vi "log_data.vi"(0 "Log File":path, 1 "Carrier amplitudes":T7 format="%#_3p", 2 "Display card":i32=1 min=0 max=3 step=1, 5 "Start Logging":bool, 7 "High carrier amplitudes":T4 format="%#_3p", 9 "Stop Logging":bool, 11 "Time Stamp":timestamp, 12 "Trace info":T1, 13 "Log mode":T5, 14 "Modulation info":T6={"Fs full"=0.0, "Fs high"=0.0, "Fs low"=0.0, "Read size"=5000, "FFT size low"=5000, "df low"=5000.0, "High carriers"=[], "Low carriers"=[], "Hi channels at low"=[7]} {"Hi channels at low" min=0 step=1; "Low carriers" format="%#_6p"; "High carriers" format="%#_6p"}) -> (4 "Logging":bool)   [LabVIEW 2014]
doc: "Converts an array of data to a row of tab-separated columns, prepends the timestamp column, and terminates each row with the end of line character."
uses:
  processing/carrier_amplitudes.ctl
  processing/modulation_info.ctl
  log_mode.ctl
  processing/high_carrier_amplitudes.ctl
  gui/trace_info.ctl
  gui/trace_channel.ctl
  main/ilemt_status.ctl
  main/ilemt_globals.vi
panel:
  out "Result string":string
  # "Debug display:"
  # "Note that each dumped row is a couping matrix in column major format, where rows are source axes and columns are sensor axes. See comment in coupling_to_string for more details."
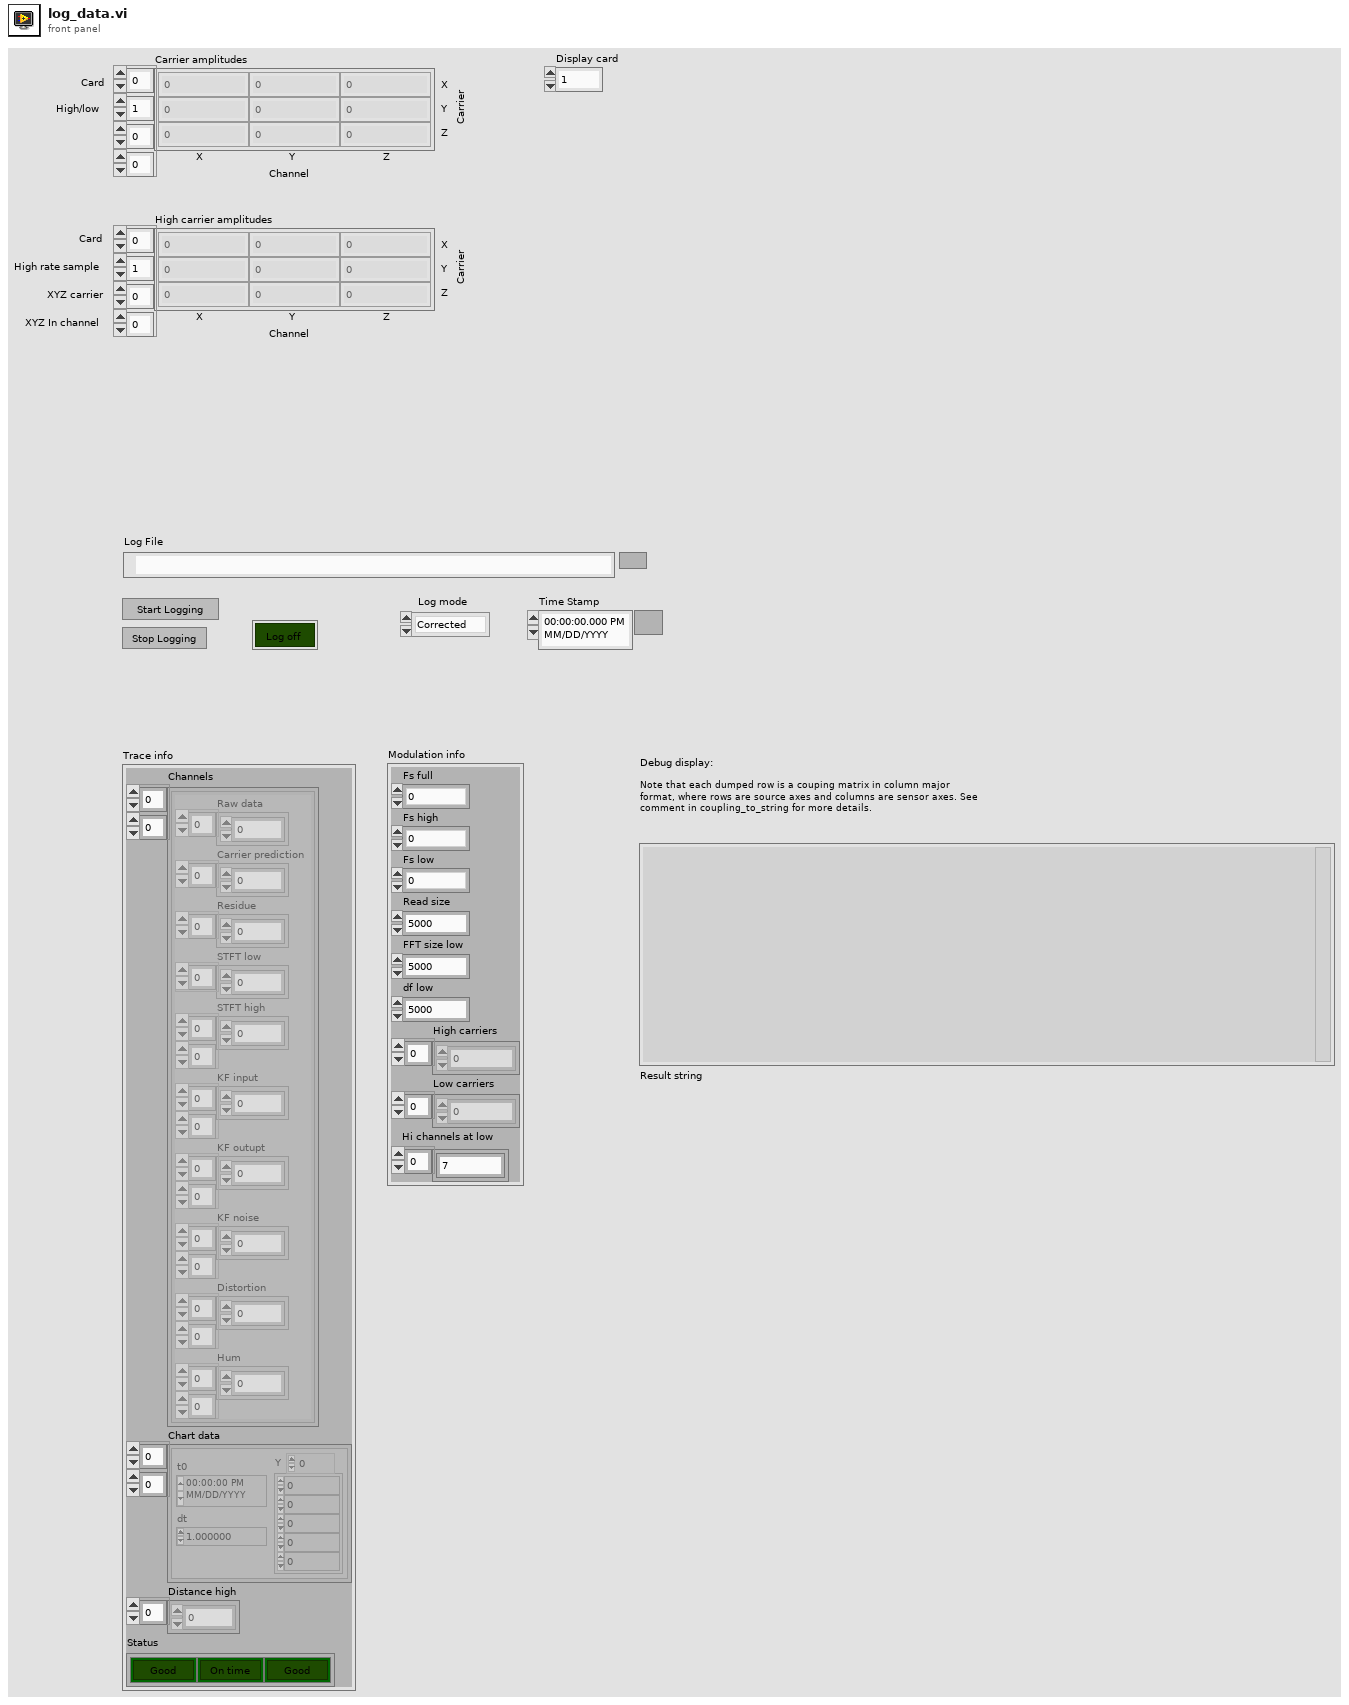
[diagram p1: front panel]
types:
  T1 = typedef "trace_info.ctl" = cluster{"Channels":T2[][], "Chart data":waveform(dbl)[][], "Distance high":dbl[], "Status":T3}
  T2 = typedef "trace_channel.ctl" = cluster{"Raw data":dbl[], "Carrier prediction":dbl[], "Residue":dbl[], "STFT low":cdb[], "STFT high":cdb[][], "KF input":cdb[][], "KF outupt":cdb[][], "KF noise":dbl[][], "Distortion":cdb[][], "Hum":cdb[][]}
  T3 = typedef "ilemt_status.ctl" = cluster{"NaN":bool, "Backlog":bool, "Clipping":bool}
  T4 = typedef "high_carrier_amplitudes.ctl" = cdb[][][][]
  T5 = typedef "log_mode.ctl" = enum16{"Corrected", "Raw"}
  T6 = typedef "modulation_info.ctl" = cluster{"Fs full":dbl, "Fs high":dbl, "Fs low":dbl, "Read size":i32, "FFT size low":i32, "df low":dbl, "High carriers":dbl[], "Low carriers":dbl[], "Hi channels at low":i32[]}
  T7 = typedef "carrier_amplitudes.ctl" = cdb[][][][]
  T8 = enum16{"open", "replace", "create", "open or create", "replace or create", "replace or create with confirmation"}
  T9 = typedef "coupling_matrix.ctl" = cdb[][]
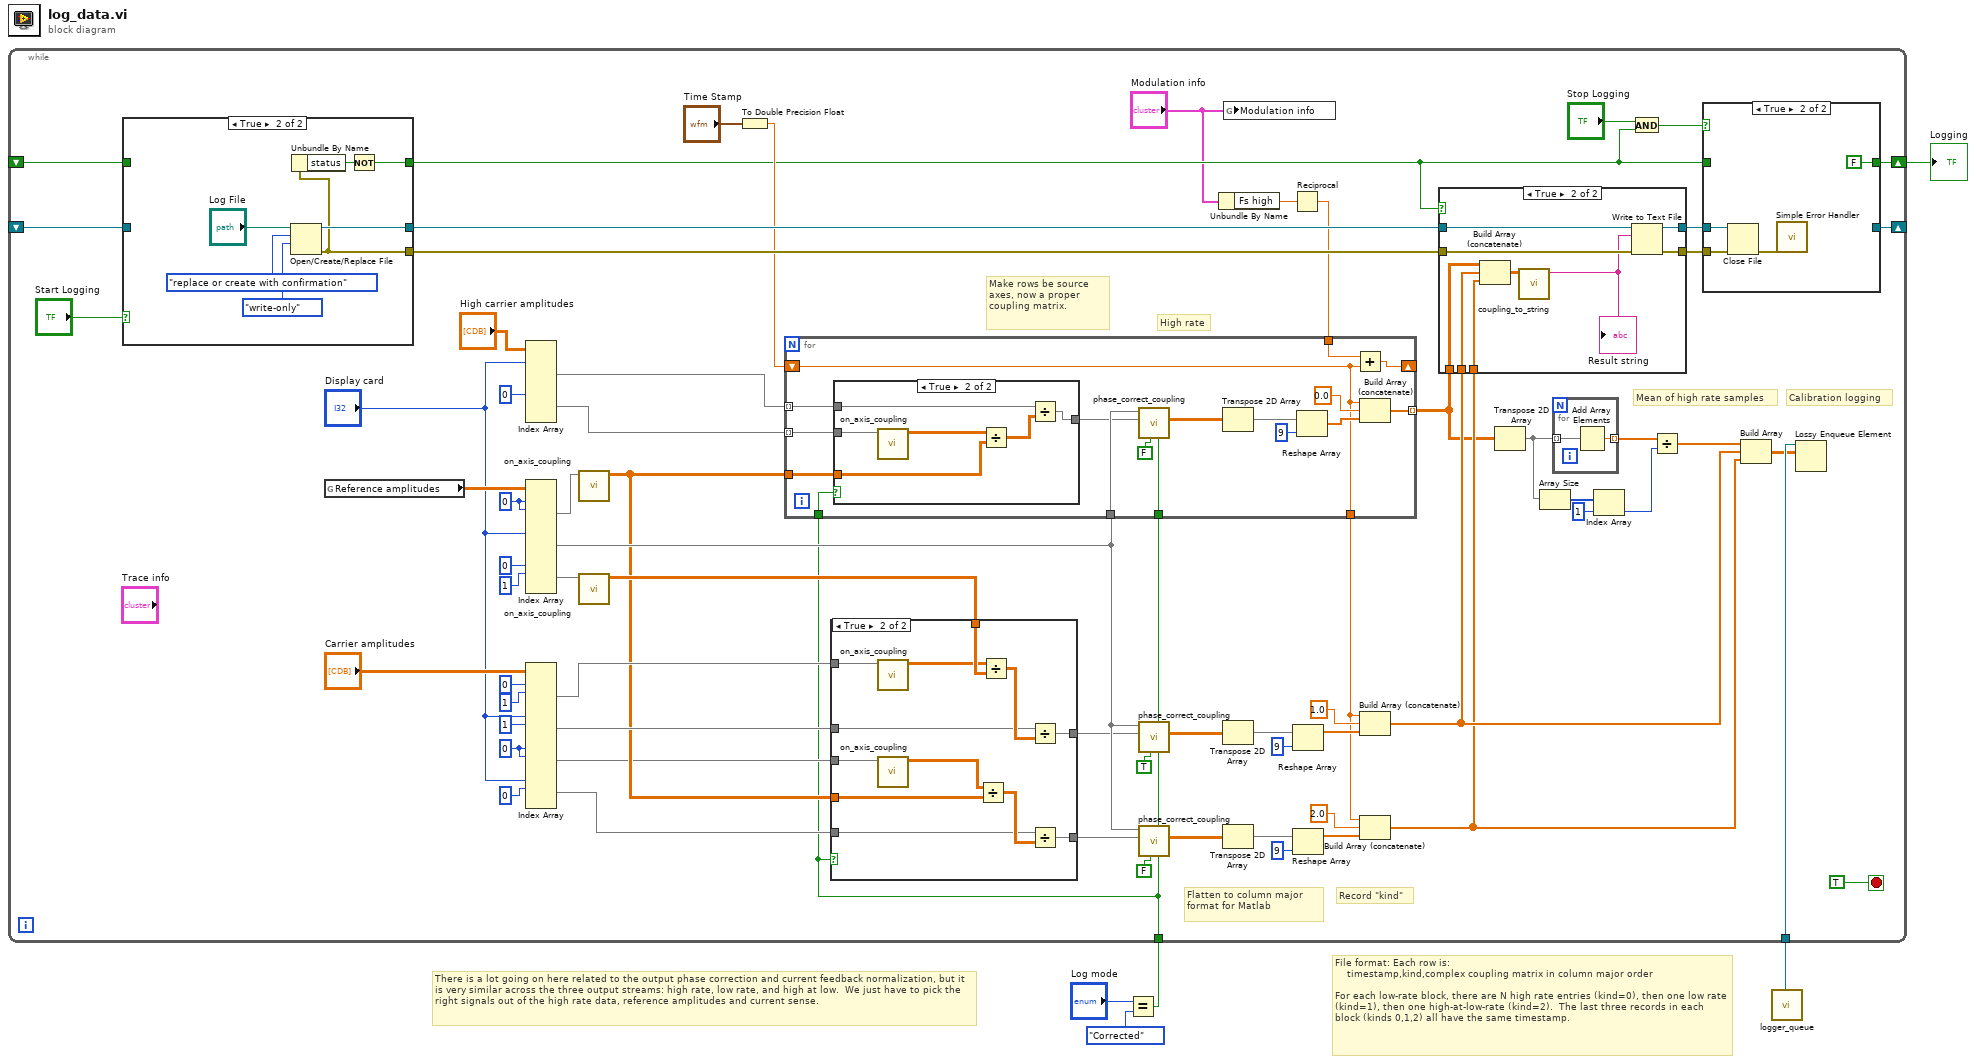
[diagram p0: block diagram]
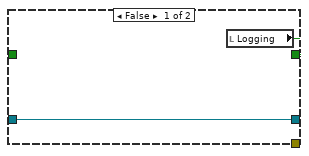
[diagram p6: hidden frame]
diagram:
  # "There is a lot going on here related to the output phase correction and current feedback normalization, but it is very similar across the three output streams: high rate, low rate, and high at low.  We just have to pick the right signals out of the high rate data, reference amplitudes and current sense."
  # "File format: Each row is:\n    timestamp,kind,complex coupling matrix in column major order\n\nFor each low-rate block, there are N high rate entries (kind=0), then one low rate (kind=1), then one high-at-low-rate (kind=2).  The last three records in each block (kinds 0,1,2) all have the same timestamp."
  n1 = Equal?(x="Log mode", y=log_mode."Corrected") -> (x = y?=w1:bool)
  n2 = call "logger_queue.vi"() -> ("queue out"=w4:refnum<queue>)  [unwired: 10 in, 1 out]
  n3 = while {
    shift-right: [w70] -> _
    shift-left: _ -> [w71]
    shift-right: [w63] -> w5
    shift-left: _ -> [w64]
    tunnel: w4 -> [w42]
    tunnel: w1 -> [w9]
    stop <- TRUE stop-if-true
    w11 = 0 ("index (vol)")
    w8 = 0 ("index (vol)")
    # "Calibration logging"
    # "Record \"kind\""
    # "Mean of high rate samples"
    # "Make rows be source axes, now a proper coupling matrix."
    # "Flatten to column major format for Matlab"
    # "High rate"
    n4 = case shown="True" "Start Logging" {
      tunnel: [w133 w140] -> w73
      tunnel: [_ w136] -> w74
      tunnel: w71 -> [w133 _]
      tunnel: [w132 w134] -> w45
      tunnel: w64 -> [_ _]
      frame False {
        n5 = local read "Logging"() -> (w132:bool)
      }
      frame True {
        n6 = Open/Create/Replace File(file path (use dialog)="Log File", operation (0:open)=T8."replace or create with confirmation", access (0:read/write)=enum16{"read/write", "read-only", "write-only"}."write-only") -> (refnum out=w140:refnum<file>, error out=w136:errorcluster)  [unwired: 2 in, 2 out]
        n7 = Unbundle By Name(w136) -> ("status"=w135:bool)
        n8 = Not(x=w135) -> (.not. x?=w134:bool)
      }
    }
    n9 = global read "ilemt_globals.vi" "Reference amplitudes"() -> (w30:T7)
    n10 = Index Array(array="High carrier amplitudes", index (dim 0) #1="Display card", index (dim 0) #2=0 ("index (vol)")) -> (element #1=w27:cdb[][][], element #2=w28:cdb[][][])  [unwired: 6 in]
    n11 = Index Array(array=w30, index (dim 0) #1=w8, index (dim 1) #1=w8, index (dim 0) #2="Display card", index (dim 0) #3=0 ("index (vol)"), index (dim 1) #3=1 ("index (page)")) -> (element #1=w31:cdb[][], element #2=w21:cdb[][][], element #3=w24:cdb[][])  [unwired: 7 in]
    n12 = Index Array(array="Carrier amplitudes", index (dim 0) #1=0 ("index (vol)"), index (dim 1) #1=1 ("index (page)"), index (dim 0) #2="Display card", index (dim 1) #2=1 ("disabled index (page)"), index (dim 0) #3=w11, index (dim 1) #3=w11, index (dim 0) #4="Display card", index (dim 1) #4=0 ("disabled index (page)")) -> (element #1=w18:cdb[][], element #2=w16:cdb[][], element #3=w10:cdb[][], element #4=w12:cdb[][])  [unwired: 8 in]
    n13 = call "on_axis_coupling.vi"("Sense coupling"=w31) -> ("Sense amplitudes"=w14:T9)  [unwired: 10 in]
    n14 = call "on_axis_coupling.vi"("Sense coupling"=w24) -> ("Sense amplitudes"=w17:T9)  [unwired: 10 in]
    n15 = To Double Precision Float(number="Time Stamp") -> (double precision float=w54:dbl)
    n16 = case shown="True" w9 {
      tunnel: w18 -> [_ w87]
      tunnel: w17 -> [_ w86]
      tunnel: w16 -> [w76 w85]
      tunnel: [w76 w84] -> w15
      tunnel: w14 -> [_ w82]
      tunnel: [w75 w81] -> w13
      tunnel: w12 -> [w75 w79]
      tunnel: w10 -> [_ w78]
      frame False {
      }
      frame True {
        n17 = call "on_axis_coupling.vi"("Sense coupling"=w87) -> ("Sense amplitudes"=w83:T9)  [unwired: 10 in]
        n18 = call "on_axis_coupling.vi"("Sense coupling"=w78) -> ("Sense amplitudes"=w77:T9)  [unwired: 10 in]
        n19 = Divide(x=w77, y=w82) -> (x/y=w80:T9)
        n20 = Divide(x=w83, y=w86) -> (x/y=w88:T9)
        n21 = Divide(x=w85, y=w88) -> (x/y=w84:cdb[][])
        n22 = Divide(x=w79, y=w80) -> (x/y=w81:cdb[][])
      }
    }
    n23 = call "phase_correct_coupling.vi"("Really correct?"=w9, "Is low?"=TRUE, "Complex coupling"=w15, "Ref carrier ampl"=w21) -> ("Phase corrected coupling"=w58:cdb[][])  [unwired: 6 in, 1 out]
    n24 = call "phase_correct_coupling.vi"("Really correct?"=w9, "Is low?"=FALSE, "Complex coupling"=w13, "Ref carrier ampl"=w21) -> ("Phase corrected coupling"=w51:cdb[][])  [unwired: 6 in, 1 out]
    n25 = Unbundle By Name("Modulation info") -> ("Fs high"=w56:dbl)
    n26 = Transpose 2D Array(2D array=w58) -> (transposed array=w57:cdb[][])
    n27 = Transpose 2D Array(2D array=w51) -> (transposed array=w52:cdb[][])
    n28 = global write "ilemt_globals.vi" "Modulation info"("Modulation info") -> ()
    n29 = Reciprocal(x=w56) -> (1/x=w53:dbl)
    n30 = for {
      tunnel: [w114] -> w37 mode=indexing
      tunnel: w21 -> [w107]
      shift-right: [w112] -> _
      shift-left: w54 -> [w110]
      tunnel: w53 -> [w113]
      tunnel: [w110] -> w46
      tunnel: w9 -> [w111]
      tunnel: w28 -> [w106] mode=indexing
      tunnel: w14 -> [w105]
      tunnel: w27 -> [w104] mode=indexing
      tunnel: w9 -> [w102]
      n31 = case shown="True" w102 {
        tunnel: w106 -> [_ w124]
        tunnel: w105 -> [_ w123]
        tunnel: w104 -> [w119 w122]
        tunnel: [w119 w120] -> w103
        frame False {
        }
        frame True {
          n32 = call "on_axis_coupling.vi"("Sense coupling"=w124) -> ("Sense amplitudes"=w125:T9)  [unwired: 10 in]
          n33 = Divide(x=w125, y=w123) -> (x/y=w121:T9)
          n34 = Divide(x=w122, y=w121) -> (x/y=w120:cdb[][])
        }
      }
      n35 = call "phase_correct_coupling.vi"("Really correct?"=w111, "Is low?"=FALSE, "Complex coupling"=w103, "Ref carrier ampl"=w107) -> ("Phase corrected coupling"=w109:cdb[][])  [unwired: 6 in, 1 out]
      n36 = Transpose 2D Array(2D array=w109) -> (transposed array=w108:cdb[][])
      n37 = Reshape Array(w108, 9 ("dimension size")) -> (w116:cdb[])
      n38 = Add(x=w113, y=w110) -> (x+y=w112:dbl)
      n39 = Build Array (concatenate)(w110, 0.0, w116) -> (w114:cdb[])
    }
    n40 = Reshape Array(w57, 9 ("dimension size")) -> (w61:cdb[])
    n41 = Reshape Array(w52, 9 ("dimension size")) -> (w48:cdb[])
    n42 = Build Array (concatenate)(w46, 1.0, w61) -> (w44:cdb[])
    n43 = Build Array (concatenate)(w46, 2.0, w48) -> (w43:cdb[])
    n44 = case shown="True" w45 {
      tunnel: w74 -> [w91 w101]
      tunnel: w73 -> [w92 w100]
      tunnel: [w92 w99] -> w69
      tunnel: [w91 w98] -> w68
      tunnel: w44 -> [_ w97]
      tunnel: w37 -> [_ w96]
      tunnel: w43 -> [_ w93]
      frame False {
      }
      frame True {
        n45 = Build Array (concatenate)(w96, w97, w93) -> (w95:cdb[][])
        n46 = call "coupling_to_string.vi"("Coupling data"=w95) -> ("Result string"=w94:string)  [unwired: 10 in]
        "Result string" <- w94
        n47 = Write to Text File(file (use dialog)=w100, text=w94, error in=w101) -> (refnum out=w99:refnum<file>, error out=w98:errorcluster)  [unwired: 1 in, 1 out]
      }
    }
    n48 = Transpose 2D Array(2D array=w37) -> (transposed array=w33:cdb[][])
    n49 = Array Size(array=w33) -> (size(s)=w36:i32[])
    n50 = for {
      tunnel: w33 -> [w90] mode=indexing
      tunnel: [w89] -> w38 mode=indexing
      n51 = Add Array Elements(numeric array=w90) -> (sum=w89:cdb)
    }
    n52 = Index Array(array=w36, index=1) -> (element=w34:i32)
    n53 = And(x="Stop Logging", y=w45) -> (x .and. y?=w67:bool)
    n54 = Divide(x=w38, y=w34) -> (x/y=w39:cdb[])
    n55 = case shown="True" w67 {
      tunnel: [w127 _] -> w70
      tunnel: w69 -> [w127 w130]
      tunnel: w68 -> [_ w129]
      tunnel: [w126 FALSE] -> w63
      tunnel: w45 -> [w126 _]
      frame False {
      }
      frame True {
        n56 = Close File(refnum=w130, error in=w129) -> (error out=w131:errorcluster)  [unwired: 1 out]
        n57 = call <vilib>:"Simple Error Handler.vi"("error in (no error)"=w131) -> ()  [unwired: 1 in, 8 out]
      }
    }
    n58 = Build Array(w39, w44, w43) -> (w41:cdb[][])
    n59 = Lossy Enqueue Element(queue=w42, element=w41) -> ()  [unwired: 1 in, 4 out]
  }
  "Logging" <- w5
